vi "Handle getAll.vi"(8 "error in (no error)":errorcluster, 11 "Inst.Krohn-Hite-7008 in":refnum<class "Inst.Krohn-Hite-7008.lvclass">) -> (0 "error out":errorcluster, 2 "getAll":variant, 3 "Inst.Krohn-Hite-7008 out":refnum<class "Inst.Krohn-Hite-7008.lvclass">)   [LabVIEW 2019, in "Inst.KH7008.lvlib" / "Inst.Krohn-Hite-7008.lvclass"]
uses:
  Inst.Krohn-Hite-7008.lvclass
  Inst.Krohn-Hite-7008.lvclass/Inst.Krohn-Hite-7008.ctl
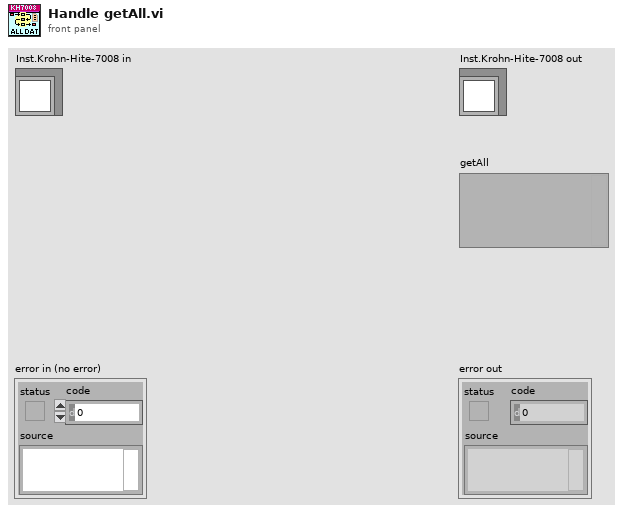
[diagram p1: front panel]
types:
  T1 = typedef "Inst.KH7008.lvlib/Inst.Krohn-Hite-7008.lvclass/Inst.Krohn-Hite-7008.getAll--Cluster.ctl" = cluster{"allChannelProperties":T2}
  T2 = typedef "KH7008.lvlib/allChannelProperties--Array.ctl" = T3[]
  T3 = typedef "KH7008.lvlib/channelProperties--Cluster.ctl" = cluster{"channel":T4, "gain":T5, "input":T6, "shunt":T7, "couple":T8, "filter":T9}
  T4 = typedef "KH7008.lvlib/channel--numeric.ctl" = u16
  T5 = typedef "KH7008.lvlib/gain--enum.ctl" = enum16{"1", "10", "100", "1000"}
  T6 = typedef "KH7008.lvlib/input--enum.ctl" = enum16{"OFF", "SE+", "SE-", "DIFF"}
  T7 = typedef "KH7008.lvlib/shunt--enum.ctl" = enum16{"Open", "50", "500", "5k", "50k", "10M"}
  T8 = typedef "KH7008.lvlib/couple--enum.ctl" = enum16{"AC", "DC"}
  T9 = typedef "KH7008.lvlib/filter--enum.ctl" = enum16{"OFF", "ON"}
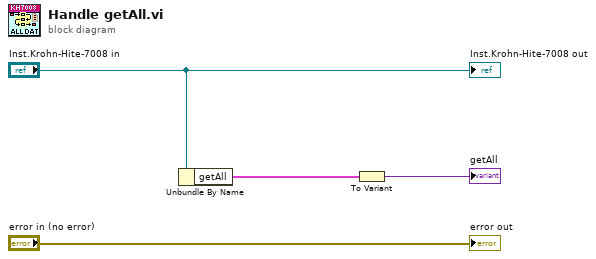
[diagram p0: block diagram]
diagram:
  n1 = Unbundle By Name("Inst.Krohn-Hite-7008 in") -> ("getAll"=w4:T1)
  n2 = To Variant(anything=w4) -> (Variant=→"getAll":variant)
  "error out" <- "error in (no error)"
  "Inst.Krohn-Hite-7008 out" <- "Inst.Krohn-Hite-7008 in"
